vi "InitDC.vi"(8 "error in (no error)":errorcluster, 11 "DataCollector in":refnum<class "DataCollector.lvclass">) -> (0 "error out":errorcluster, 3 "DataCollector out":refnum<class "DataCollector.lvclass">)   [LabVIEW 2017, in "DataCollector.lvclass"]
uses:
  DataCollector.lvclass
  DataCollector.lvclass/DataCollector.ctl
  <vilib>/drjdpowell/SQLite Library/SQL Connection/Execute SQL (Single Integer).vi
  <vilib>/drjdpowell/SQLite Library/SQLite.lvlib
  <vilib>/drjdpowell/SQLite Library/SQL Connection/Connection.lvclass
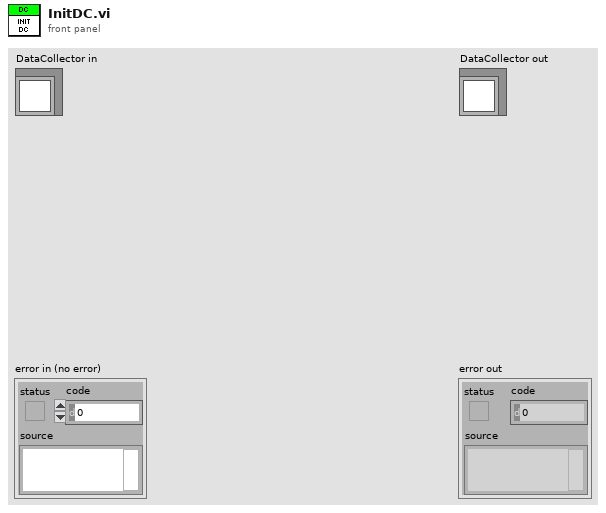
[diagram p1: front panel]
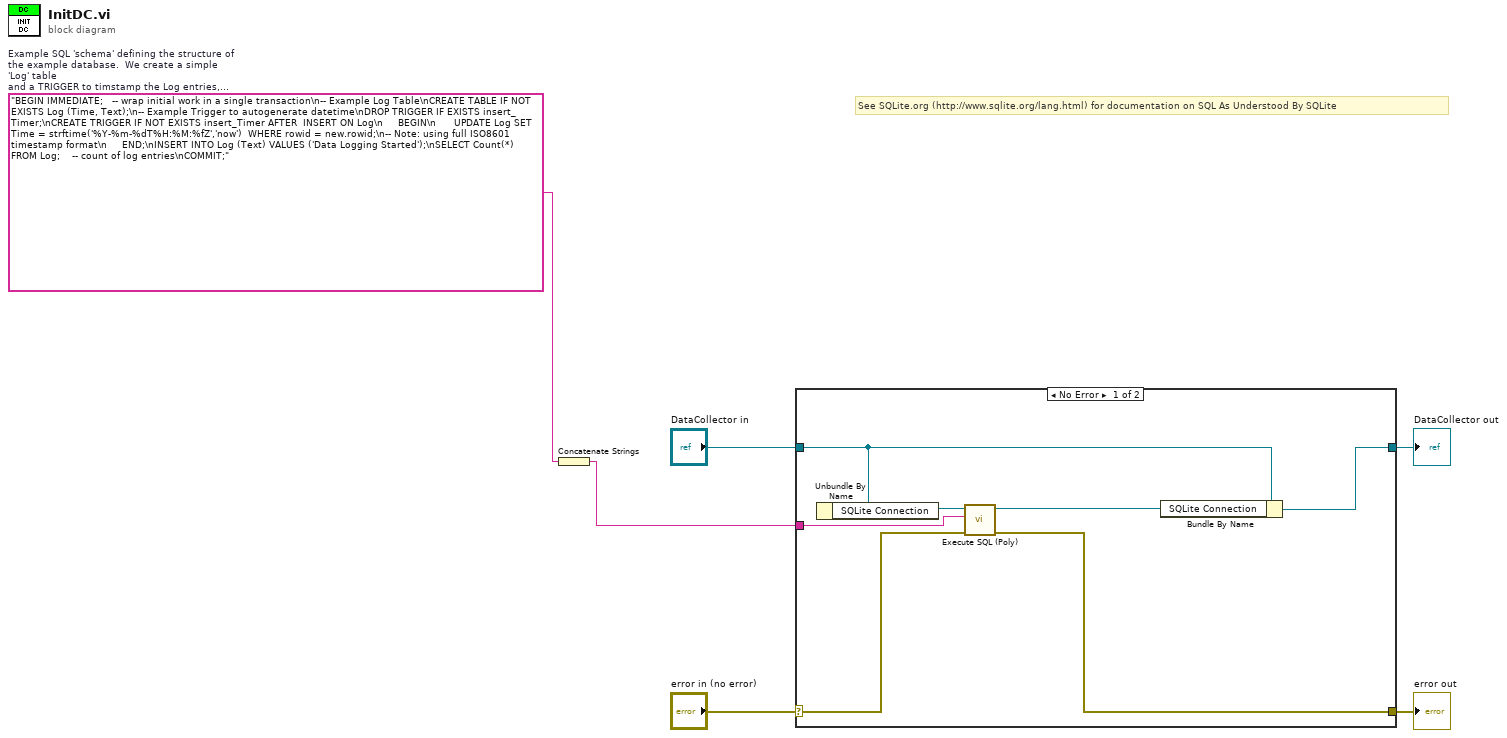
[diagram p0: block diagram]
diagram:
  w2 = "BEGIN IMMEDIATE;   -- wrap initial work in a single transaction\n-- Example Log Table\nCREATE TABLE IF NOT EXISTS Log (Time, Text);\n-- Example Trigger to autogenerate datetime\nDROP TRIGGER IF EXISTS insert_Timer;\nCREATE TRIGGER IF NOT EXISTS insert_Timer AFTER  INSERT ON Log\n     BEGIN\n      UPDATE Log SET Time = strftime('%Y-%m-%dT%H:%M:%fZ','now')  WHERE rowid = new.rowid;\n-- Note: using full ISO8601 timestamp format\n     END;\nINSERT INTO Log (Text) VALUES ('Data Logging Started');\nSELECT Count(*) FROM Log;    -- count of log entries\nCOMMIT;"  # Example SQL 'schema' defining the structure of the example database.  We create a simple 'Log' table and a TRIGGER to timstamp the Log entries, then a simple 'Data' table
  # "See SQLite.org (http://www.sqlite.org/lang.html) for documentation on SQL As Understood By SQLite"
  n1 = Concatenate Strings(w2) -> (w1:string)
  n2 = case shown="No Error" "error in (no error)" {
    selector: "error in (no error)" -> [w9 w15]
    tunnel: [w8 w15] -> w5
    tunnel: [w11 w14] -> w3
    tunnel: "DataCollector in" -> [w12 w14]
    tunnel: w1 -> [w7 _]
    frame No Error {
      n3 = Unbundle By Name(w12) -> ("SQLite Connection"=w13:refnum<class "Connection.lvclass">)
      n4 = call-poly <vilib>:"Execute SQL (Poly).vi"("error in (no error)"=w9, "SQL"=w7, "SQLite Connection in"=w13) -> ("error out"=w8:errorcluster, "SQLite Connection out"=w10:refnum<class "Connection.lvclass">)  [unwired: 6 in, 1 out]
      n5 = Bundle By Name(cluster=w12, "SQLite Connection"=w10) -> (w11:refnum<class "DataCollector.lvclass">)
    }
    frame Error {
    }
  }
  "error out" <- w5
  "DataCollector out" <- w3
